vi "perpheralsInitialise.vi"(8 "Edge Axis Labels only":bool, 9 "Cols":u8, 10 "Rows":u8, 11 "GraphPeripheralsIn":T1[][](array[typedef])) -> (3 "GraphPeripheralsOut":T1[][](array[typedef]))   [LabVIEW 2012]
uses:
  graphPeripherals.ctl
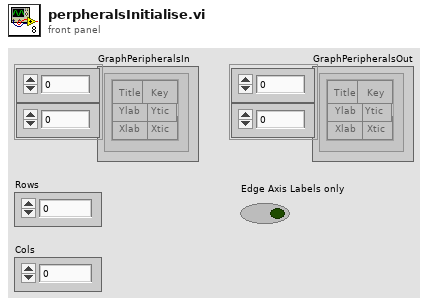
[diagram p1: front panel]
types:
  T1 = typedef "graphPeripherals.ctl" = cluster{"title":bool, "key":bool, "Xtic":bool, "Ytic":bool, "Xlab":bool, "Ylab":bool}
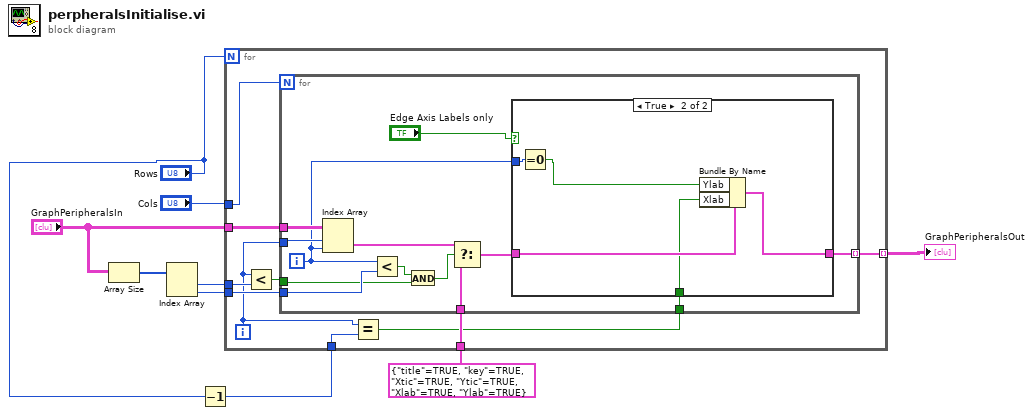
[diagram p0: block diagram]
diagram:
  n1 = Array Size(array="GraphPeripheralsIn") -> (size(s)=w6:i32[])
  n2 = Index Array(array=w6) -> (element #1=w7:i32, element #2=w8:i32)  [unwired: 2 in]
  n3 = Decrement(x="Rows") -> (x-1=w1:u8)
  n4 = for {
    N: "Rows" -> [_]
    tunnel: "Cols" -> [w19]
    tunnel: "GraphPeripheralsIn" -> [w18]
    tunnel: [w17] -> w3 mode=indexing
    tunnel: w7 -> [w16]
    tunnel: w8 -> [w15]
    tunnel: T1 {"title"=TRUE, "key"=TRUE, "Xtic"=TRUE, "Ytic"=TRUE, "Xlab"=TRUE, "Ylab"=TRUE} ("Peripherals") -> [w13]
    tunnel: w1 -> [w12]
    i -> [w11]
    n5 = Less?(x=w11, y=w16) -> (x < y?=w14:bool)
    n6 = Equal?(x=w11, y=w12) -> (x = y?=w10:bool)
    n7 = for {
      N: w19 -> [_]
      tunnel: w18 -> [w32]
      tunnel: w11 -> [w31]
      tunnel: [w23] -> w17 mode=indexing
      tunnel: w15 -> [w30]
      tunnel: w14 -> [w28]
      tunnel: w13 -> [w25]
      tunnel: w10 -> [w20]
      i -> [w21]
      n8 = Index Array(array=w32, index (row)=w31, index (col)=w21) -> (element=w26:T1)
      n9 = Less?(x=w21, y=w30) -> (x < y?=w29:bool)
      n10 = And(x=w29, y=w28) -> (x .and. y?=w27:bool)
      n11 = Select(t=w26, s=w27, f=w25) -> (s? t:f=w22:T1)
      n12 = case shown="True" "Edge Axis Labels only" {
        tunnel: [w33 w36] -> w23
        tunnel: w22 -> [w33 w37]
        tunnel: w21 -> [_ w38]
        tunnel: w20 -> [_ w34]
        frame False {
        }
        frame True {
          n13 = Equal To 0?(x=w38) -> (x = 0?=w35:bool)
          n14 = Bundle By Name(cluster=w37, "Ylab"=w35, "Xlab"=w34) -> (w36:T1)
        }
      }
    }
  }
  "GraphPeripheralsOut" <- w3
